vi "NXT_HINDBRAIN ESTOP.vi"(3 "Hard E-Stop":bool, 4 "_sensorData":T1, 5 "_fromPC":u8[](array[numeric])) -> (0 "Soft E-Stop":bool, 1 "Hard E-Stop":bool)   [LabVIEW 2012, in "Tugboat.lvrbt"]
uses:
  Tugboat.lvrbt
  sensorData_t.ctl
  irData_t.ctl
panel:
  # "L\nE\nF\nT"
  # "C\nE\nN\nT\nE\nR"
  # "R\nI\nG\nH\nT"
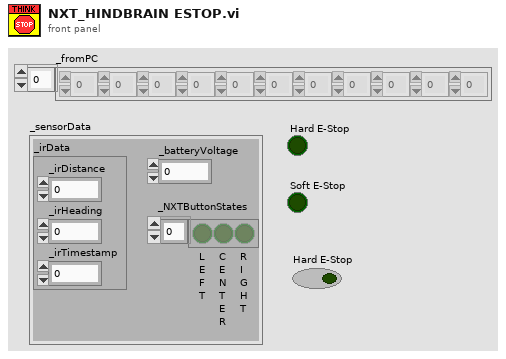
[diagram p1: front panel]
types:
  T1 = typedef "sensorData_t.ctl" = cluster{"_irData":T2, "_batteryVoltage":i32, "_NXTButtonStates":bool[]}
  T2 = typedef "irData_t.ctl" = cluster{"_irDistance":i32, "_irHeading":i32, "_irTimestamp":u32}
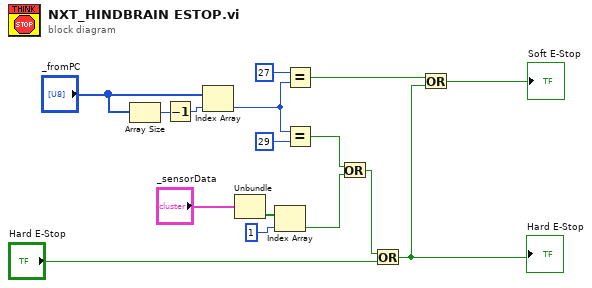
[diagram p0: block diagram]
diagram:
  n1 = Array Size(array="_fromPC") -> (size(s)=w13:i32)
  n2 = Decrement(x=w13) -> (x-1=w12:i32)
  n3 = Index Array(array="_fromPC", index=w12) -> (element=w11:u8)
  n4 = Unbundle("_sensorData") -> ("_NXTButtonStates"=w14:bool[])  [unwired: 2 out]
  n5 = Index Array(array=w14, index=1) -> (element=w7:bool)
  n6 = Equal?(x=u8 27, y=w11) -> (x = y?=w2:bool)
  n7 = Equal?(x=w11, y=u8 29) -> (x = y?=w8:bool)
  n8 = Or(x=w8, y=w7) -> (x .or. y?=w5:bool)
  n9 = Or(x=w5, y="Hard E-Stop") -> (x .or. y?=w4:bool)
  "Hard E-Stop" <- w4
  n10 = Or(x=w2, y=w4) -> (x .or. y?=→"Soft E-Stop":bool)
